vi "Port table.vi"() -> (0 "Port table":T1[](array[typedef])=[{"Name"="bnc_panel.ai0", "Line"="Dev3/ai0"}, {"Name"="bnc_panel.ai1", "Line"="Dev3/ai1"}, {"Name"="bnc_panel.ai2", "Line"="Dev3/ai2"}, {"Name"="bnc_panel.ai3", "Line"="Dev3/ai3"}, {"Name"="bnc_panel.ai4", "Line"="Dev3/ai4"}, {"Name"="bnc_panel.ai5", "Line"="Dev3/ai5"}, {"Name"="bnc_panel.ai6", "Line"="Dev3/ai6"}, {"Name"="bnc_panel.ai7", "Line"="Dev3/ai7"}, {"Name"="bnc_panel.p0.0", "Line"="Dev3/port0/line0"}, {"Name"="bnc_panel.p0.1", "Line"="Dev3/port0/line1"}, {"Name"="bnc_panel.p0.2", "Line"="Dev3/port0/line2"}, {"Name"="bnc_panel.p0.3", "Line"="Dev3/port0/line3"}, {"Name"="bnc_panel.p0.4", "Line"="Dev3/port0/line4"}, {"Name"="bnc_panel.p0.5", "Line"="Dev3/port0/line5"}, {"Name"="bnc_panel.p0.6", "Line"="Dev3/port0/line6"}, {"Name"="bnc_panel.p0.7", "Line"="Dev3/port0/line7"}, {"Name"="bnc_panel.p1.0", "Line"="Dev3/port1/line0"}, {"Name"="bnc_panel.p1.1", "Line"="Dev3/port1/line1"}, {"Name"="bnc_panel.p1.2", "Line"="Dev3/port1/line2"}, {"Name"="bnc_panel.p1.3", "Line"="Dev3/port1/line3"}, {"Name"="bnc_panel.p1.4", "Line"="Dev3/port1/line4"}, {"Name"="bnc_panel.p1.5", "Line"="Dev3/port1/line5"}, {"Name"="bnc_panel.p1.6", "Line"="Dev3/port1/line6"}, {"Name"="bnc_panel.p1.7", "Line"="Dev3/port1/line7"}, {"Name"="juicer.valve1", "Line"="Dev2/port0/line0"}, {"Name"="juicer.valve2", "Line"="Dev2/port0/line1"}, {"Name"="juicer.valve3", "Line"="Dev2/port0/line2"}, {"Name"="juicer.valve4", "Line"="Dev2/port0/line3"}, {"Name"="juicer.valve5", "Line"="Dev2/port0/line4"}, {"Name"="juicer.valve6", "Line"="Dev2/port0/line5"}, {"Name"="juicer.valve7", "Line"="Dev2/port1/line0"}, {"Name"="juicer.valve8", "Line"="Dev2/port1/line1"}, {"Name"="juicer.valve9", "Line"="Dev2/port1/line2"}, {"Name"="juicer.valve10", "Line"="Dev2/port1/line3"}, {"Name"="juicer.valve11", "Line"="Dev2/port1/line4"}, {"Name"="juicer.valve12", "Line"="Dev2/port1/line5"}, {"Name"="juicer.flush", "Line"="Dev2/port1/line6"}, {"Name"="juicer.purge", "Line"="Dev2/port1/line7"}, {"Name"="juicer.bleed1", "Line"="Dev2/port0/line6"}, {"Name"="juicer.bleed2", "Line"="Dev2/port0/line7"}, {"Name"="Dsub_panel.P9.7", "Line"="Dev2/port9/line7"}, {"Name"="bnc_panel.ao0", "Line"="Dev3/ao0"}, {"Name"="bnc_panel.ao1", "Line"="Dev3/ao1"}, {"Name"="bnc_panel.ao2", "Line"="Dev3/ao2"}, {"Name"="bnc_panel.ao3", "Line"="Dev3/ao3"}, {"Name"="beam.1", "Line"="Dev2/port5/line0"}, {"Name"="beam.2", "Line"="Dev2/port2/line5"}, {"Name"="beam.3", "Line"="Dev2/port5/line2"}, {"Name"="beam.4", "Line"="Dev2/port5/line3"}, {"Name"="beam.5", "Line"="Dev2/port5/line4"}, {"Name"="beam.6", "Line"="Dev2/port5/line6"}, {"Name"="beam.7", "Line"="Dev2/port2/line3"}, {"Name"="beam.8", "Line"="Dev2/port2/line1"}, {"Name"="beam.11", "Line"="Dev2/port2/line4"}, {"Name"="beam.12", "Line"="Dev2/port5/line1"}, {"Name"="beam.13", "Line"="Dev2/port2/line0"}, {"Name"="beam.14", "Line"="Dev2/port2/line2"}, {"Name"="beam.15", "Line"="Dev2/port5/line5"}, {"Name"="beam.not_a_real_beam", "Line"="Dev2/port2/line6"}, {"Name"="door.1", "Line"="Dev2/port3/line2"}, {"Name"="door.2", "Line"="Dev2/port3/line0"}, {"Name"="door.3", "Line"="Dev2/port3/line7"}, {"Name"="door.4", "Line"="Dev2/port3/line1"}, {"Name"="door.5", "Line"="Dev2/port3/line4"}, {"Name"="door.6", "Line"="Dev2/port3/line5"}, {"Name"="door.7", "Line"="Dev2/port3/line6"}, {"Name"="door.8", "Line"="Dev2/port3/line3"}])   [LabVIEW 2015]
uses:
  Rack/Typedefs/Port table entry.ctl
panel:
  in  "Tab Control":enum32{"Setup", "Nothing to see here"}(tab)
  in  "Port table setup":T1[](array[typedef])=[{"Name"="bnc_panel.ai0", "Line"="Dev3/ai0"}, {"Name"="bnc_panel.ai1", "Line"="Dev3/ai1"}, {"Name"="bnc_panel.ai2", "Line"="Dev3/ai2"}, {"Name"="bnc_panel.ai3", "Line"="Dev3/ai3"}, {"Name"="bnc_panel.ai4", "Line"="Dev3/ai4"}, {"Name"="bnc_panel.ai5", "Line"="Dev3/ai5"}, {"Name"="bnc_panel.ai6", "Line"="Dev3/ai6"}, {"Name"="bnc_panel.ai7", "Line"="Dev3/ai7"}, {"Name"="bnc_panel.p0.0", "Line"="Dev3/port0/line0"}, {"Name"="bnc_panel.p0.1", "Line"="Dev3/port0/line1"}, {"Name"="bnc_panel.p0.2", "Line"="Dev3/port0/line2"}, {"Name"="bnc_panel.p0.3", "Line"="Dev3/port0/line3"}, {"Name"="bnc_panel.p0.4", "Line"="Dev3/port0/line4"}, {"Name"="bnc_panel.p0.5", "Line"="Dev3/port0/line5"}, {"Name"="bnc_panel.p0.6", "Line"="Dev3/port0/line6"}, {"Name"="bnc_panel.p0.7", "Line"="Dev3/port0/line7"}, {"Name"="bnc_panel.p1.0", "Line"="Dev3/port1/line0"}, {"Name"="bnc_panel.p1.1", "Line"="Dev3/port1/line1"}, {"Name"="bnc_panel.p1.2", "Line"="Dev3/port1/line2"}, {"Name"="bnc_panel.p1.3", "Line"="Dev3/port1/line3"}, {"Name"="bnc_panel.p1.4", "Line"="Dev3/port1/line4"}, {"Name"="bnc_panel.p1.5", "Line"="Dev3/port1/line5"}, {"Name"="bnc_panel.p1.6", "Line"="Dev3/port1/line6"}, {"Name"="bnc_panel.p1.7", "Line"="Dev3/port1/line7"}, {"Name"="juicer.valve1", "Line"="Dev2/port0/line0"}, {"Name"="juicer.valve2", "Line"="Dev2/port0/line1"}, {"Name"="juicer.valve3", "Line"="Dev2/port0/line2"}, {"Name"="juicer.valve4", "Line"="Dev2/port0/line3"}, {"Name"="juicer.valve5", "Line"="Dev2/port0/line4"}, {"Name"="juicer.valve6", "Line"="Dev2/port0/line5"}, {"Name"="juicer.valve7", "Line"="Dev2/port1/line0"}, {"Name"="juicer.valve8", "Line"="Dev2/port1/line1"}, {"Name"="juicer.valve9", "Line"="Dev2/port1/line2"}, {"Name"="juicer.valve10", "Line"="Dev2/port1/line3"}, {"Name"="juicer.valve11", "Line"="Dev2/port1/line4"}, {"Name"="juicer.valve12", "Line"="Dev2/port1/line5"}, {"Name"="juicer.flush", "Line"="Dev2/port1/line6"}, {"Name"="juicer.purge", "Line"="Dev2/port1/line7"}, {"Name"="juicer.bleed1", "Line"="Dev2/port0/line6"}, {"Name"="juicer.bleed2", "Line"="Dev2/port0/line7"}, {"Name"="Dsub_panel.P9.7", "Line"="Dev2/port9/line7"}, {"Name"="bnc_panel.ao0", "Line"="Dev3/ao0"}, {"Name"="bnc_panel.ao1", "Line"="Dev3/ao1"}, {"Name"="bnc_panel.ao2", "Line"="Dev3/ao2"}, {"Name"="bnc_panel.ao3", "Line"="Dev3/ao3"}, {"Name"="beam.1", "Line"="Dev2/port5/line0"}, {"Name"="beam.2", "Line"="Dev2/port2/line5"}, {"Name"="beam.3", "Line"="Dev2/port5/line2"}, {"Name"="beam.4", "Line"="Dev2/port5/line3"}, {"Name"="beam.5", "Line"="Dev2/port5/line4"}, {"Name"="beam.6", "Line"="Dev2/port5/line6"}, {"Name"="beam.7", "Line"="Dev2/port2/line3"}, {"Name"="beam.8", "Line"="Dev2/port2/line1"}, {"Name"="beam.11", "Line"="Dev2/port2/line4"}, {"Name"="beam.12", "Line"="Dev2/port5/line1"}, {"Name"="beam.13", "Line"="Dev2/port2/line0"}, {"Name"="beam.14", "Line"="Dev2/port2/line2"}, {"Name"="beam.15", "Line"="Dev2/port5/line5"}, {"Name"="beam.not_a_real_beam", "Line"="Dev2/port2/line6"}, {"Name"="door.1", "Line"="Dev2/port3/line2"}, {"Name"="door.2", "Line"="Dev2/port3/line0"}, {"Name"="door.3", "Line"="Dev2/port3/line7"}, {"Name"="door.4", "Line"="Dev2/port3/line1"}, {"Name"="door.5", "Line"="Dev2/port3/line4"}, {"Name"="door.6", "Line"="Dev2/port3/line5"}, {"Name"="door.7", "Line"="Dev2/port3/line6"}, {"Name"="door.8", "Line"="Dev2/port3/line3"}]
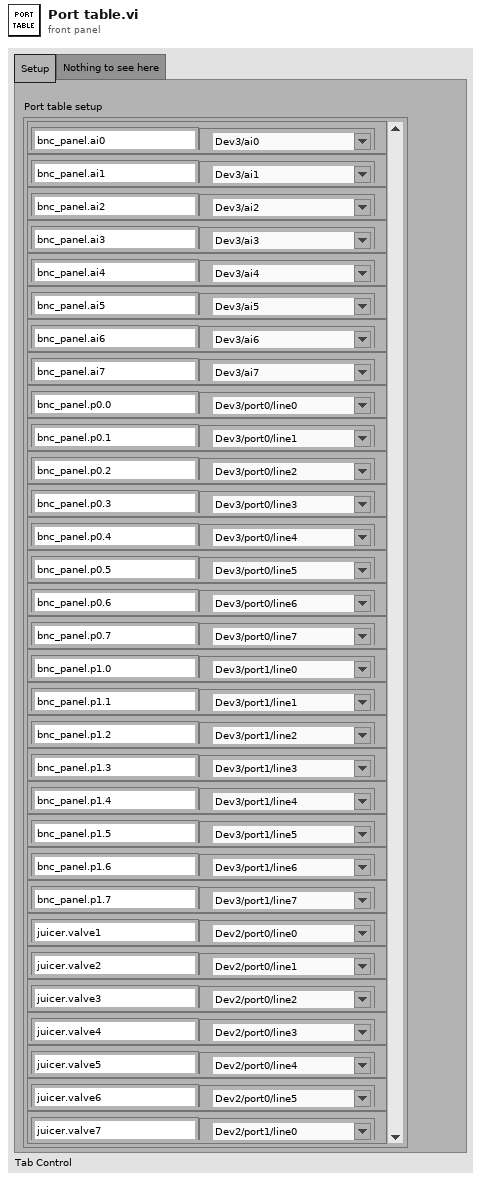
[diagram p1: front panel]
types:
  T1 = typedef "Port table entry.ctl" = cluster{"Name":string, "Line":tag}
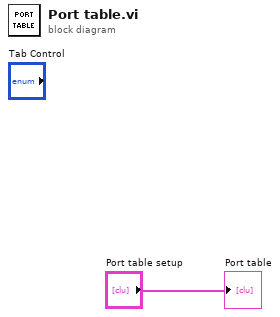
[diagram p0: block diagram]
diagram:
  "Port table" <- "Port table setup"
